vi "Data_Get Time.vi"(8 "error in (no error)":errorcluster, 11 "variant":variant) -> (0 "error out":errorcluster, 1 "Last Start Time":timestamp, 3 "variant out":variant)   [LabVIEW 2015, in "Exposure Process.lvlib"]
uses:
  Exposure Process.lvlib
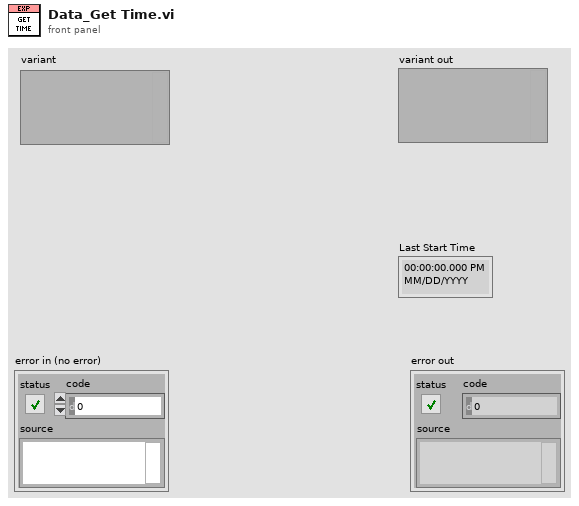
[diagram p1: front panel]
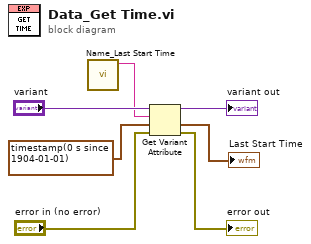
[diagram p0: block diagram]
diagram:
  n1 = call "Name_Last Start Time.vi"() -> ("Name"=w6:string)  [unwired: 11 in]
  n2 = Get Variant Attribute(Variant="variant", name=w6, default value (empty Variant)=timestamp(0 s since 1904-01-01), error in="error in (no error)") -> (duplicate Variant=→"variant out":variant, value=→"Last Start Time":timestamp, error out=→"error out":errorcluster)  [unwired: 1 out]
